vi "test_ThreeSessThreePinTwoInstrTwoSiteReservation_CallGetConnectionsFromPinsForPinNameWithWrongCase_ReturnsError.vi"(8 "error in":errorcluster) -> (0 "error out":errorcluster, 2 "result":string, 3 "pass":bool)   [LabVIEW 2020, in "MeasurementServerTests.lvlib"]
uses:
  MeasurementServerTests.lvlib
  Runtime/APIs/Session Management V1/Session Reservation/Connection.ctl
  Runtime/APIs/Session Management V1/Session Reservation/Session Reservation.lvclass
  Runtime/APIs/Session Management V1/Session Reservation/Connection with Session.ctl
  c3cb69a0-23cd-49fc-99d1-8c54773f0200.vi
  Runtime/Measurements/Helpers/Error Strings Global Internal.vi
  Runtime/Sessions/niDCPower Sessions/Session Factory/Session Factory.lvclass
  Runtime/APIs/Session Management V1/Session Reservation/Pin Type.ctl
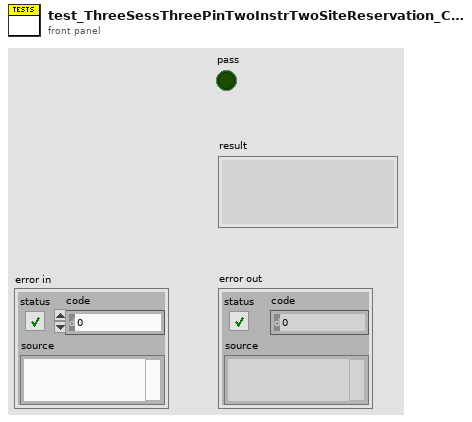
[diagram p1: front panel]
types:
  T1 = typedef "Plug-In SDK Session Management V1.lvlib/Session Reservation.lvclass/Pin Type.ctl" = enum16{"DUT and System Pins", "System Pins"}
  T2 = typedef "Plug-In SDK Session Management V1.lvlib/Session Reservation.lvclass/Connection with Session.ctl" = cluster{"connection":T3, "session":variant}
  T3 = typedef "Plug-In SDK Session Management V1.lvlib/Session Reservation.lvclass/Connection.ctl" = cluster{"pin or relay name":string, "site":i32, "instrument type id":string, "channel":string}
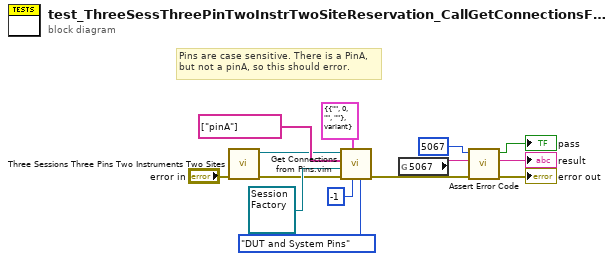
[diagram p0: block diagram]
diagram:
  # "Pins are case sensitive. There is a PinA,\nbut not a pinA, so this should error."
  n1 = call "Three Sessions Three Pins Two Instruments Two Sites.vi"("error in"="error in") -> ("error out"=w2:errorcluster, "session reservation out"=w1:refnum<class "Session Reservation.lvclass">)  [unwired: 8 in, 1 out]
  n2 = call "Get Connections from Pins.vim"("pin type"=Pin_Type."DUT and System Pins", "site"=-1, "connection type"=T2 {"connection"={"pin or relay name"="", "site"=0, "instrument type id"="", "channel"=""}, "session"=variant} ("connection"), "error in"=w2, "session factory"=refnum<class "Session Factory.lvclass"> refnum ("MeasurementLink niDCPower.lvlib:Instrument.lvclass"), "pin or relay names"=string[] ["pinA"], "session reservation in"=w1) -> ("error out"=w8:errorcluster)  [unwired: 2 in, 2 out]
  n3 = global read "Error Strings Global Internal.vi" "5067"() -> (w9:string)
  n4 = call "Assert Error Code.vi"("error in"=w8, "expected error description"=w9, "expected error code"=5067) -> ("error out"=→"error out":errorcluster, "details"=→"result":string, "error code match?"=→"pass":bool)  [unwired: 6 in]
